vi "OBJ_MAIN_history_listbox_alternate_colors.vi"(6 "Recolor? (T)":bool=TRUE, 8 "error_in":errorcluster, 10 "item_names":string[][](array[string]), 11 "listbox_ref":refnum<vi>) -> (0 "error_out":errorcluster)   [LabVIEW 2019]
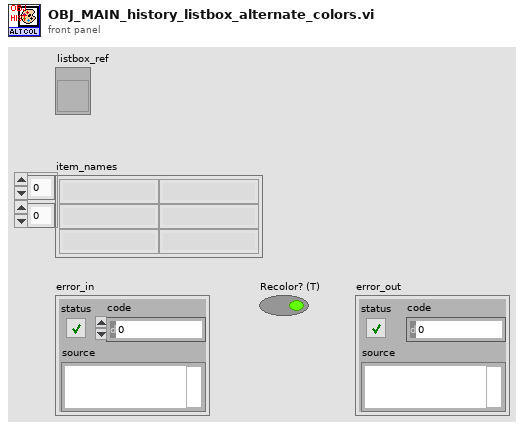
[diagram p1: front panel]
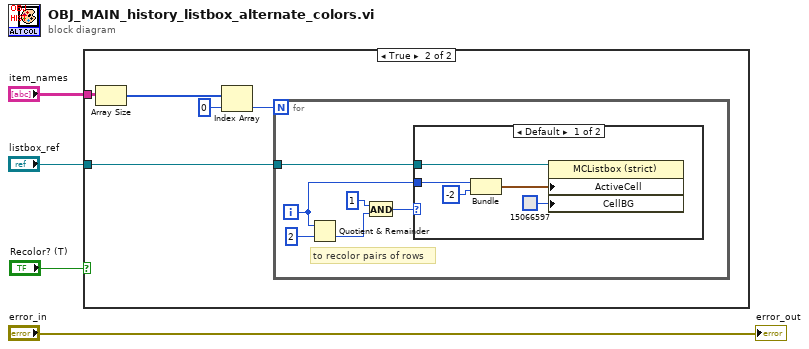
[diagram p0: block diagram]
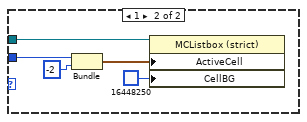
[diagram p3: hidden frame]
diagram:
  n1 = case shown="True" "Recolor? (T)" {
    tunnel: "item_names" -> [_ w6]
    tunnel: "listbox_ref" -> [_ w5]
    frame False {
    }
    frame True {
      n2 = Array Size(array=w6) -> (size(s)=w7:i32[])
      n3 = Index Array(array=w7, index=0) -> (element=w8:i32)
      n4 = for {
        N: w8 -> [_]
        tunnel: w5 -> [w15]
        i -> [w10]
        # "to recolor pairs of rows"
        n5 = Quotient & Remainder(x=w10, y=2) -> (floor(x/y)=w11:i32)  [unwired: 1 out]
        n6 = And(x=1, y=w11) -> (x .and. y?=w14:i32)
        n7 = case shown="Default" w14 {
          tunnel: w15 -> [w20 w24]
          tunnel: w10 -> [w16 w25]
          frame Default {
            n8 = Bundle(w16, -2) -> (w18:cluster{i32, i32})  [unwired: 1 in]
            n9 = property on="Property Node" class="MCListbox (strict)"(reference=w20, "ActiveCell"=w18, "CellBG"=u32 15066597) -> ()  [unwired: 1 in, 2 out]
          }
          frame 1 {
            n10 = Bundle(w25, -2) -> (w22:cluster{i32, i32})  [unwired: 1 in]
            n11 = property on="Property Node" class="MCListbox (strict)"(reference=w24, "ActiveCell"=w22, "CellBG"=u32 16448250) -> ()  [unwired: 1 in, 2 out]
          }
        }
      }
    }
  }
  "error_out" <- "error_in"
